vi "Create.vi"(7 "Sender":refnum<class "Sender.lvclass">, 9 "jettl":refnum<class "jettl.lvclass">, 10 "Self Alias":string, 11 "TEMPLATE jettl in":refnum<class "TEMPLATE jettl.lvclass">) -> (3 "TEMPLATE jettl out":refnum<class "TEMPLATE jettl.lvclass">)   [LabVIEW 2021, in "_Template.lvlib" / "Templates.lvlib" / "TEMPLATE jettl.lvlib" / "TEMPLATE jettl.lvclass"]
uses:
  TEMPLATE jettl.lvclass
  TEMPLATE jettl.lvclass/TEMPLATE jettl.ctl
  jettl/jettl/jettl/jettl.lvclass
  jettl/jettl/Sender/Sender/Sender.lvclass
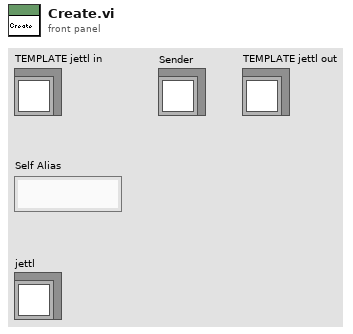
[diagram p1: front panel]
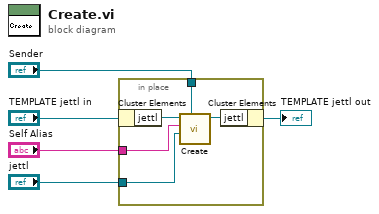
[diagram p0: block diagram]
diagram:
  n1 = in-place {
    in-place-border: "Self Alias" -> [w8]
    in-place-border: "jettl" -> [w7]
    in-place-border: "Sender" -> [w6]
    n2 = in-place-cluster #1("TEMPLATE jettl in") -> ("jettl"=w10:refnum<class "jettl.lvclass">)
    n3 = call-dynamic "Create.vi"("Sender"=w6, "jettl"=w7, "Self Alias"=w8, "Create in"=w10) -> ("Create out"=w9:refnum<class "jettl.lvclass">)  [unwired: 7 in]
    n4 = in-place-cluster #1("jettl"=w9) -> (→"TEMPLATE jettl out":refnum<class "TEMPLATE jettl.lvclass">)
  }
